vi "Test Device by Resource.vi"() -> ()   [LabVIEW 2020]
uses:
  Device/Device Info.ctl
  VisaResource/VisaResource.lvclass
  C:/dev/Vireo/PicoG/PicoG-Processor/PicoG-Core/DeployResource/DeployResource.lvclass
  DeviceManager.lvclass
  Device/Device.lvclass
panel:
  out "error out":errorcluster
  out "Array":T1[](array[typedef])
  in  "Resource":refnum<visa-resource-name>
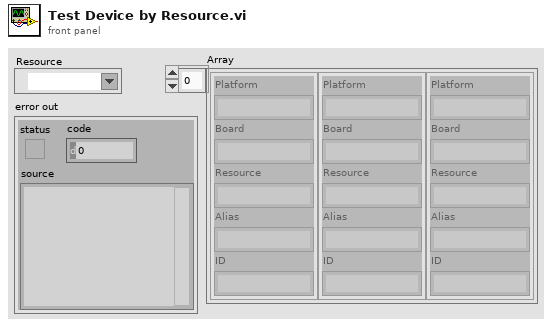
[diagram p1: front panel]
types:
  T1 = typedef "PicoG-Core.lvlib/Device.lvclass/Device Info.ctl" = cluster{"Platform":string, "Board":string, "Resource":string, "Alias":string, "ID":string}
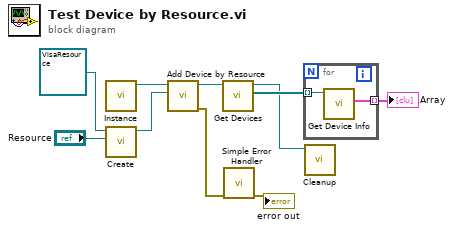
[diagram p0: block diagram]
diagram:
  n1 = call "Instance.vi"() -> ("Device Manager"=w8:refnum<class "DeviceManager.lvclass">)  [unwired: 10 in, 1 out]
  n2 = call-dynamic "Create.vi"("Resource"="Resource", "VisaResource in"=refnum<class "VisaResource.lvclass"> refnum) -> ("VisaResource out"=w7:refnum<class "VisaResource.lvclass">)  [unwired: 8 in, 1 out]
  n3 = call "Add Device by Resource.vi"("Resource"=w7, "DeviceManager in"=w8) -> ("error out"=w2:errorcluster, "DeviceManager out"=w6:refnum<class "DeviceManager.lvclass">)  [unwired: 7 in, 1 out]
  n4 = call "Get Devices.vi"("DeviceManager in"=w6) -> ("Devices"=w5:refnum<class "Device.lvclass">[], "DeviceManager out"=w3:refnum<class "DeviceManager.lvclass">)  [unwired: 8 in, 1 out]
  n5 = call <vilib>:"Simple Error Handler.vi"("error in (no error)"=w2) -> ("error out"=→"error out":errorcluster)  [unwired: 4 in, 4 out]
  n6 = for {
    tunnel: w5 -> [w12] mode=indexing
    tunnel: [w11] -> w4 mode=indexing
    n7 = call "Get Device Info.vi"("Device in"=w12) -> ("Device Info"=w11:T1)  [unwired: 8 in, 2 out]
  }
  "Array" <- w4
  n8 = call "Cleanup.vi"("DeviceManager in"=w3) -> ()  [unwired: 10 in, 1 out]
